vi "InitNetworkImpairParams.vi"(8 "ErrorArray In":errorcluster[](array[cluster])) -> (0 "ErrorArray Out":errorcluster[](array[cluster]))   [LabVIEW 2014, in "Framework.lvlib"]
uses:
  Framework.lvlib
  TypeDefs/clInitParams.ctl
  <vilib>/Utility/error.llb/Error Cluster From Error Code.vi
  <vilib>/ErrorRing/Error Ring.xnode
  <vilib>/Utility/config.llb/NI_LVConfig.lvlib
  <userlib>/NIST/NISTErrorLib/NISTErrorLib.lvlib
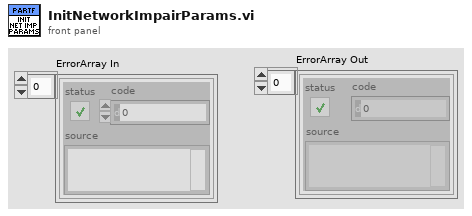
[diagram p1: front panel]
types:
  T1 = typedef "Framework.lvlib/clFrontPanelControlRefs.ctl" = cluster{"TestFilePathRef":refnum<vi>, "BusNumberRef":refnum<vi>, "NumberOfBusesRef":refnum<vi>, "EvtTypeRef":refnum<vi>, "EvtParamsRef":refnum<vi>, "EvtConfigRef":refnum<vi>, "StartTimeRef":refnum<vi>, "EndTimeRef":refnum<vi>, "PmuImpairTypeRef":refnum<vi>, "PmuImpairParamsRef":refnum<vi>, "NetImpairParamsRef":refnum<vi>, "FlagImpairTypeRef":refnum<vi>, "FlagImpairParamsRef":refnum<vi>, "NetImpairTypeRef":refnum<vi>, "OutputFileType":refnum<vi>, "PmuImpairConfigRef":refnum<vi>, "AppTypeRef":refnum<vi>, "ScriptPathRef":refnum<vi>, "ShowPanels?":refnum<vi>}
  T2 = typedef "Framework.lvlib/clInitParams.ctl" = cluster{"RowHdrs":string[], "ColHdrs":string[], "DefaultParams":string[][]}
  T3 = typedef "Framework.lvlib/clFrameworkData.ctl" = cluster{"EvtINIFilePaths":path[], "BusClassInstances":refnum<class "Bus.lvclass">[], "PmuImpairINIFilePaths":path[], "FlagImpairINIFilePaths":path[], "NetImpairINIFilePaths":path[], "OutputToFileINIFilePaths":path[], "AppINIFilePaths":path[], "AppModuleID":i32, "OutputToFileID":i32}
  T4 = typedef "NI_LVConfig.lvlib/Config Data RefNum.ctl" = refnum<k1>
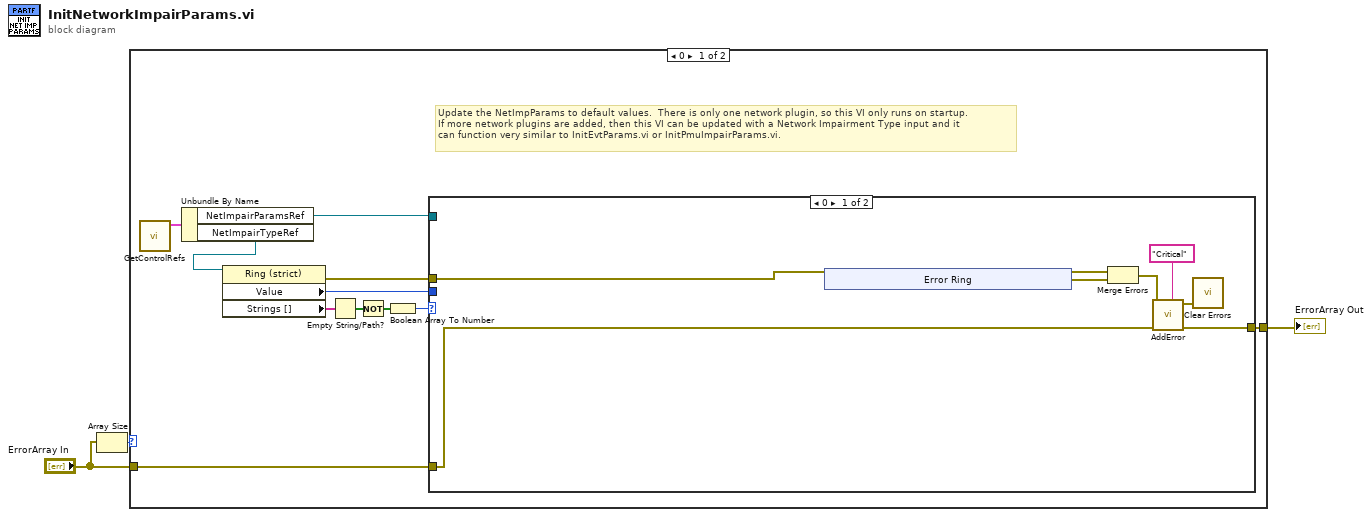
[diagram p0: block diagram]
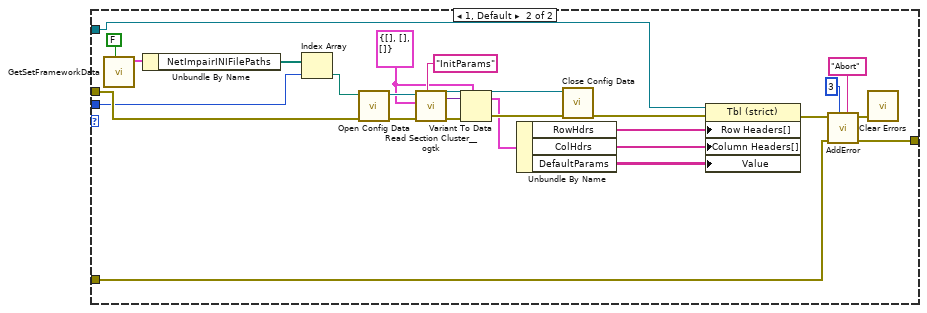
[diagram p2: hidden frame]
diagram:
  n1 = Array Size(array="ErrorArray In") -> (size(s)=w3:i32)
  n2 = case shown="0" w3 {
    tunnel: "ErrorArray In" -> [w13 w53]
    tunnel: [w12 w53] -> w1
    frame 0 {
      # "Update the NetImpParams to default values.  There is only one network plugin, so this VI only runs on startup.\nIf more network plugins are added, then this VI can be updated with a Network Impairment Type input and it\ncan function very similar to InitEvtParams.vi or InitPmuImpairParams.vi."
      n3 = call "GetControlRefs.vi"() -> ("clControlRefs Out"=w5:T1)  [unwired: 11 in]
      n4 = Unbundle By Name(w5) -> ("NetImpairParamsRef"=w14:refnum<vi>, "NetImpairTypeRef"=w4:refnum<vi>)
      n5 = property class="Ring (strict)"(reference=w4) -> (error out=w7:errorcluster, "Value"=w6:u16, "Strings []"=w9:string[])  [unwired: 1 in, 1 out]
      n6 = Empty String/Path?(string/path=w9) -> (empty?=w10:bool[])
      n7 = Not(x=w10) -> (.not. x?=w11:bool[])
      n8 = Boolean Array To Number(Boolean array=w11) -> (number=w8:u32)
      n9 = case shown="0" w8 {
        tunnel: w14 -> [_ w27]
        tunnel: w13 -> [w17 w52]
        tunnel: [w19 w51] -> w12
        tunnel: w7 -> [w15 w33]
        tunnel: w6 -> [_ w28]
        frame 0 {
          n10 = xnode "Error Ring"() -> ("error out"=w18:errorcluster)
          n11 = Merge Errors(w15, w18) -> (w16:errorcluster)
          n12 = call <userlib>:"AddError.vi"("Severity"="Critical" ("String"), "ErrorArray"=w17, "error in (no error)"=w16) -> ("ErrorArray"=w19:errorcluster[], "error out"=w20:errorcluster)  [unwired: 7 in]
          n13 = call <vilib>:"Clear Errors.vi"("error in (no error)"=w20) -> ()  [unwired: 5 in, 2 out]
        }
        frame 1, Default {
          w45 = T2 {"RowHdrs"=[], "ColHdrs"=[], "DefaultParams"=[]} ("ParamsHdrs")
          n14 = call "GetSetFrameworkData.vi"("Set (F)"=FALSE ("Set/Get")) -> ("clFrameworkData Out"=w31:T3)  [unwired: 10 in]
          n15 = Unbundle By Name(w31) -> ("NetImpairINIFilePaths"=w30:path[])
          n16 = Index Array(array=w30, index=w28) -> (element=w29:path)
          n17 = call <vilib>:"Open Config Data.vi"("error in (no error)"=w33, "configuration file path"=w29) -> ("error out"=w50:errorcluster, "refnum"=w49:T4)  [unwired: 7 in, 1 out]
          n18 = call <userlib>:"Read Section Cluster__ogtk.vi"("section (optional)"="InitParams", "error in (no error)"=w50, "Section Formatted Cluster Type"=w45, "refnum"=w49) -> ("error out"=w47:errorcluster, "Section Formatted Cluster"=w46:variant, "dup refnum"=w40:T4)  [unwired: 3 in, 2 out]
          n19 = Variant To Data(error in=w47, type=w45, Variant=w46) -> (data=w35:T2, error out=w41:errorcluster)
          n20 = Unbundle By Name(w35) -> ("RowHdrs"=w43:string[], "ColHdrs"=w44:string[], "DefaultParams"=w34:string[][])
          n21 = call <vilib>:"Close Config Data.vi"("error in (no error)"=w41, "refnum"=w40) -> ("error out"=w42:errorcluster)  [unwired: 8 in, 1 out]
          n22 = property on="Property Node" class="Tbl (strict)"(reference=w27, error in=w42, "Row Headers[]"=w43, "Column Headers[]"=w44, "Value"=w34) -> (error out=w36:errorcluster)  [unwired: 1 out]
          n23 = call <userlib>:"AddError.vi"("Severity"="Abort" ("String"), "Priority"=u8 3, "ErrorArray"=w52, "error in (no error)"=w36) -> ("ErrorArray"=w51:errorcluster[], "error out"=w37:errorcluster)  [unwired: 6 in]
          n24 = call <vilib>:"Clear Errors.vi"("error in (no error)"=w37) -> ()  [unwired: 5 in, 2 out]
        }
      }
    }
    frame 1, Default {
    }
  }
  "ErrorArray Out" <- w1
